vi "Draw Button Picture.vi"(6 "Background Color":u32(colorbox)=11776947, 7 "Button Size":i32, 8 "error in (no error)":errorcluster, 9 "Button State":T2=enum."Hover", 10 "image data":T3, 11 "Button Style":T1=enum."Classic") -> (0 "error out":errorcluster, 2 "Image (no button)":picture, 3 "Picture Out":picture)   [LabVIEW 2018, in "Button.lvclass"]
doc: "Given data about the button image, its state and overall button style, assembles a picture of the button."
uses:
  Button.lvclass
  Toolbar.xctl
  <vilib>/picture/picture.llb/imagedata.ctl
  Type Defs/Button Status.ctl
  Type Defs/Button Style.ctl
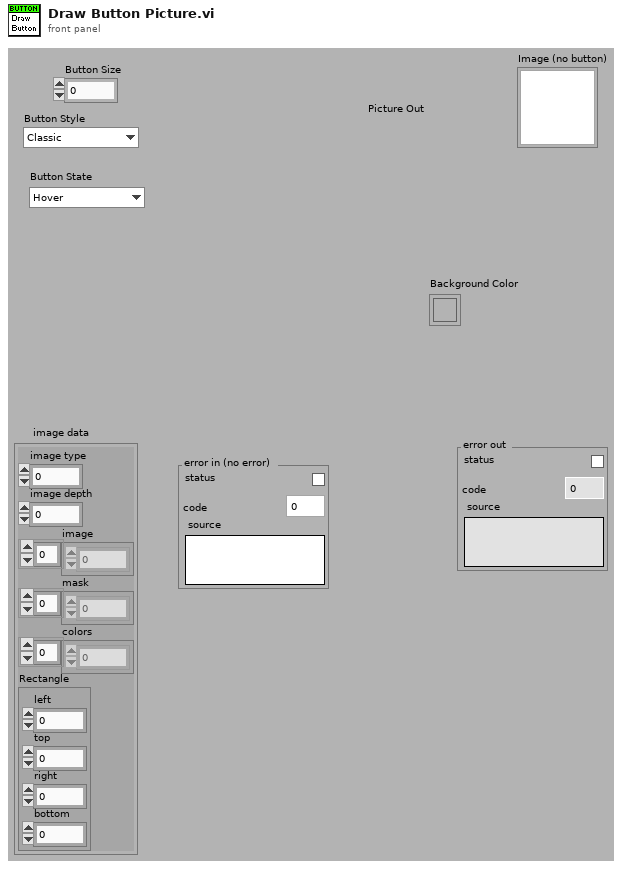
[diagram p1: front panel]
types:
  T1 = typedef "Button.lvclass/Button Style.ctl" = enum16{"System", "Modern", "Classic", "Rounded", "Silver", "Ni Theme", "Metallic"}
  T2 = typedef "Button.lvclass/Button Status.ctl" = enum16{"Off", "Hover", "On", "Disabled"}
  T3 = typedef "imagedata.ctl" = cluster{"image type":i32, "image depth":i32, "image":u8[], "mask":u8[], "colors":u32[], "Rectangle":cluster{"left":i16, "top":i16, "right":i16, "bottom":i16}}
  T4 = cluster{"left":i16, "top":i16, "right":i16, "bottom":i16}
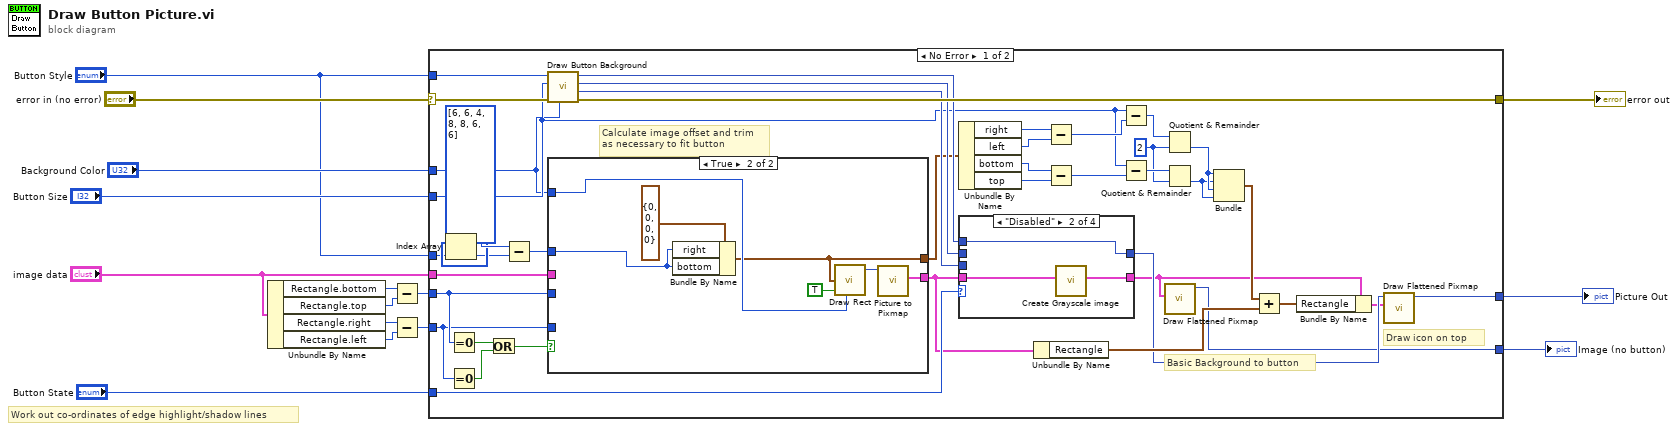
[diagram p0: block diagram]
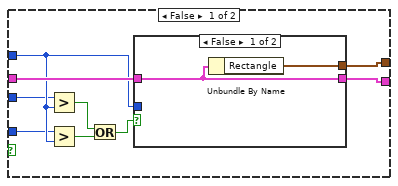
[diagram p2: hidden frame]
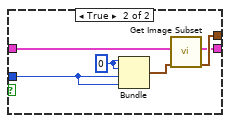
[diagram p3: hidden frame]
diagram:
  # "Work out co-ordinates of edge highlight/shadow lines"
  n1 = Unbundle By Name("image data") -> ("Rectangle.bottom"=w14:i16, "Rectangle.top"=w13:i16, "Rectangle.right"=w12:i16, "Rectangle.left"=w11:i16)
  n2 = Subtract(x=w14, y=w13) -> (x-y=w10:i16)
  n3 = Subtract(x=w12, y=w11) -> (x-y=w9:i16)
  n4 = case shown="No Error" "error in (no error)" {
    selector: "error in (no error)" -> [w48 w89]
    tunnel: "Button Size" -> [w25 _]
    tunnel: w10 -> [w24 _]
    tunnel: w9 -> [w23 _]
    tunnel: "image data" -> [w40 _]
    tunnel: "Background Color" -> [w19 _]
    tunnel: "Button State" -> [w52 _]
    tunnel: [w49 _] -> w5
    tunnel: [w47 w89] -> w4
    tunnel: "Button Style" -> [w43 _]
    tunnel: [w41 _] -> w3
    tunnel: "Button Style" -> [w17 _]
    frame No Error {
      w32 = 2 ("y")
      # "Draw icon on top"
      # "Basic Background to button"
      # "Calculate image offset and trim\nas necessary to fit button"
      n5 = Index Array(array=i32[] [6, 6, 4, 8, 8, 6, 6], index=w17) -> (element=w16:i32)
      n6 = Equal To 0?(x=w24) -> (x = 0?=w21:bool)
      n7 = Equal To 0?(x=w23) -> (x = 0?=w22:bool)
      n8 = Or(x=w21, y=w22) -> (x .or. y?=w20:bool)
      n9 = Subtract(x=w25, y=w16) -> (x-y=w28:i32)
      n10 = call "Draw Button Background.vi"("Button Color"=w19, "error in (no error)"=w48, "Button Size"=w25, "Button Style"=w43) -> ("error out"=w47:errorcluster, "On Picture"=w44:picture, "Hover Picture"=w45:picture, "Off Picture"=w46:picture)  [unwired: 4 out]
      n11 = case shown="True" w20 {
        tunnel: w40 -> [w64 _]
        tunnel: [w63 w75] -> w39
        tunnel: [w62 w74] -> w31
        tunnel: w28 -> [w61 w76]
        tunnel: w24 -> [w57 _]
        tunnel: w23 -> [w56 _]
        tunnel: w19 -> [_ w78]
        frame False {
          n12 = Greater?(x=w57, y=w61) -> (0:w60:bool)
          n13 = Greater?(x=w56, y=w61) -> (0:w59:bool)
          n14 = Or(x=w60, y=w59) -> (x .or. y?=w58:bool)
          n15 = case shown="False" w58 {
            tunnel: w61 -> [_ w72]
            tunnel: w64 -> [w66 w69]
            tunnel: [w65 w68] -> w63
            tunnel: [w66 w67] -> w62
            frame False {
              n16 = Unbundle By Name(w66) -> ("Rectangle"=w65:T4)
            }
            frame True {
              w71 = 0
              n17 = Bundle(w71, w71, w72, w72) -> (w70:cluster{i32, i32, i32, i32})  [unwired: 1 out]
              n18 = call <vilib>:"Get Image Subset.vi"("subset rect"=w70, "image data"=w69) -> ("true subset rect"=w68:T4, "image subset"=w67:T3)  [unwired: 4 out]
            }
          }
        }
        frame True {
          n19 = Bundle By Name(cluster=T4 {"left"=0, "top"=0, "right"=0, "bottom"=0} ("rect"), "right"=w76, "bottom"=w76) -> (w75:T4)
          n20 = call <vilib>:"Draw Rect.vi"("rect"=w75, "fill?(F)"=TRUE, "color(black)"=w78) -> ("new picture"=w73:picture)  [unwired: 2 in, 4 out]
          n21 = call <vilib>:"Picture to Pixmap.vi"("picture"=w73) -> ("image data"=w74:T3)  [unwired: 3 in, 7 out]
        }
      }
      n22 = Unbundle By Name(w39) -> ("right"=w38:i16, "left"=w37:i16, "bottom"=w36:i16, "top"=w35:i16)
      n23 = case shown="\"Disabled\"" w52 {
        tunnel: [w80 w82 w85 w87] -> w51
        tunnel: w31 -> [w81 w84 w86 w88]
        tunnel: [w81 w83 w86 w88] -> w42
        tunnel: w46 -> [w80 w82 _ _]
        tunnel: w45 -> [_ _ w85 _]
        tunnel: w44 -> [_ _ _ w87]
        frame "Off", Default {
        }
        frame "Disabled" {
          n24 = call "Create Grayscale image.vi"("image data"=w84) -> ("Gray scale Image"=w83:T3)  [unwired: 10 out]
        }
        frame "Hover" {
        }
        frame "On" {
        }
      }
      n25 = Unbundle By Name(w31) -> ("Rectangle"=w55:T4)
      n26 = Subtract(x=w38, y=w37) -> (x-y=w27:i16)
      n27 = Subtract(x=w36, y=w35) -> (x-y=w26:i16)
      n28 = Subtract(x=w25, y=w27) -> (x-y=w34:i32)
      n29 = Subtract(x=w25, y=w26) -> (x-y=w33:i32)
      n30 = Quotient & Remainder(x=w34, y=w32) -> (floor(x/y)=w30:i32)  [unwired: 1 out]
      n31 = Quotient & Remainder(x=w33, y=w32) -> (floor(x/y)=w29:i32)  [unwired: 1 out]
      n32 = call <vilib>:"Draw Flattened Pixmap.vi"("image data"=w42) -> ("new picture"=w41:picture)  [unwired: 1 in, 7 out]
      n33 = Bundle(w30, w29, w30, w29) -> (w54:cluster{i32, i32, i32, i32})  [unwired: 1 out]
      n34 = Add(x=w54, y=w55) -> (x+y=w53:cluster{i32, i32, i32, i32})
      n35 = Bundle By Name(cluster=w42, "Rectangle"=w53) -> (w50:T3)
      n36 = call <vilib>:"Draw Flattened Pixmap.vi"("image data"=w50, "picture"=w51) -> ("new picture"=w49:picture)  [unwired: 7 out]
    }
    frame Error {
    }
  }
  "Picture Out" <- w5
  "error out" <- w4
  "Image (no button)" <- w3
